vi "Init.vi"(8 "error in (no error)":errorcluster) -> (0 "error out":errorcluster)   [LabVIEW 2018, in "Covers-o-meter.lvlib"]
doc: "Enqueues named action and/or data."
uses:
  Covers-o-meter.lvlib
  Private/ctl/State--enum.ctl
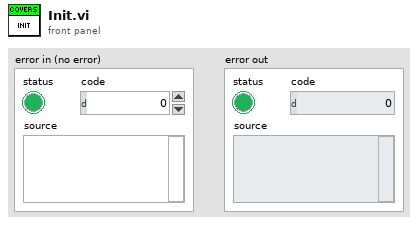
[diagram p1: front panel]
types:
  T1 = typedef "Covers-o-meter.lvlib/State--enum.ctl" = enum16{"Init", "Init: Read req tags", "Init Data: All Projects", "Init: Which Project?", "Update Requirements tags", "Get all project strings", "Search proj for tags", "Subroutine", "Update Project", "Start Button Pressed", "Start timer", "Error", "Close", "UI - Refresh Timer ", "UI - refresh graph", "UI - Refresh Tree"}
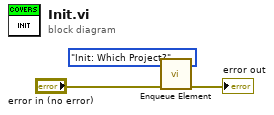
[diagram p0: block diagram]
diagram:
  n1 = call "Enqueue Element.vi"("error in"="error in (no error)", "State"=State--enum."Init: Which Project?") -> ("error out"=→"error out":errorcluster)  [unwired: 9 in]
